vi "SUM 2.vi"() -> ()   [LabVIEW 2011]
panel:
  out "0404A0EP":u8=144 format="%.0x"
  out "0404A0EN":u8=142 format="%.0x"
  out "0404A0EM":u8=203 format="%.0x"
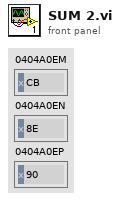
[diagram p1: front panel]
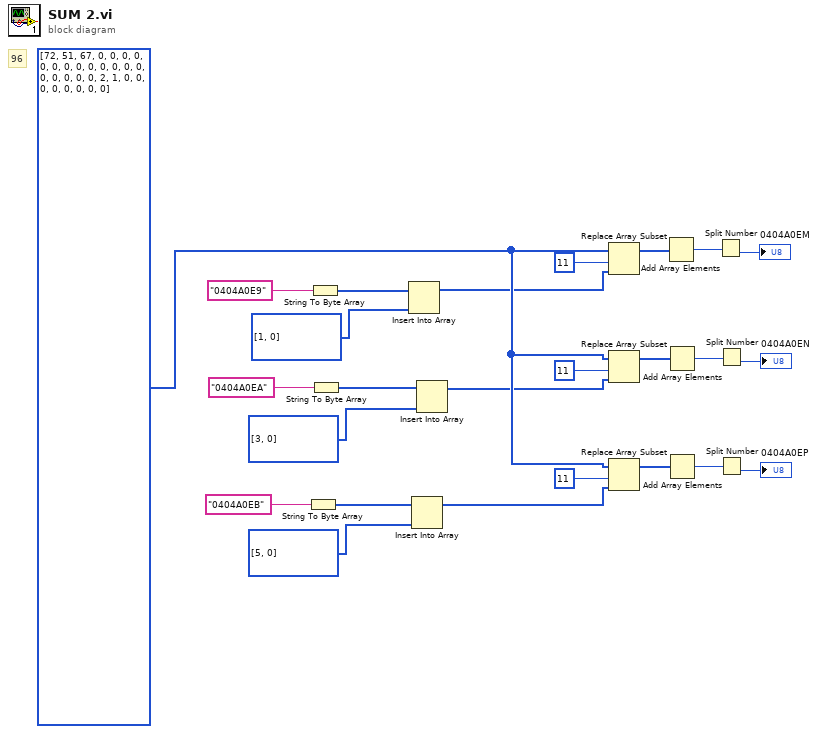
[diagram p0: block diagram]
diagram:
  w19 = u8[] [72, 51, 67, 0, 0, 0, 0, 0, 0, 0, 0, 0, 0, 0, 0, 0, 0, 0, 0, 0, 0, 2, 1, 0, 0, 0, 0, 0, 0, 0, 0] ("数组")
  # "107"
  # "126"
  # "125"
  # "120"
  # "115"
  # "116"
  # "111"
  # "110"
  # "106"
  # "105"
  # "98"
  # "101"
  # "100"
  # "96"
  n1 = String To Byte Array(string="0404A0EB") -> (unsigned byte array=w12:u8[])
  n2 = String To Byte Array(string="0404A0E9") -> (unsigned byte array=w18:u8[])
  n3 = String To Byte Array(string="0404A0EA") -> (unsigned byte array=w15:u8[])
  n4 = Insert Into Array(array=w18, new element=u8[] [1, 0] ("数组")) -> (w16:u8[])  [unwired: 1 in]
  n5 = Insert Into Array(array=w12, new element=u8[] [5, 0] ("数组")) -> (w10:u8[])  [unwired: 1 in]
  n6 = Insert Into Array(array=w15, new element=u8[] [3, 0] ("数组")) -> (w13:u8[])  [unwired: 1 in]
  n7 = Replace Array Subset(array=w19, new element=w16, index=11) -> (w9:u8[])
  n8 = Replace Array Subset(array=w19, new element=w13, index=11) -> (w8:u8[])
  n9 = Replace Array Subset(array=w19, new element=w10, index=11) -> (w7:u8[])
  n10 = Add Array Elements(numeric array=w9) -> (sum=w6:u8)
  n11 = Add Array Elements(numeric array=w8) -> (sum=w3:u8)
  n12 = Add Array Elements(numeric array=w7) -> (sum=w1:u8)
  n13 = Split Number(x=w6) -> (lo(x)=→"0404A0EM":u8)  [unwired: 1 out]
  n14 = Split Number(x=w3) -> (lo(x)=→"0404A0EN":u8)  [unwired: 1 out]
  n15 = Split Number(x=w1) -> (lo(x)=→"0404A0EP":u8)  [unwired: 1 out]
